vi "oa_Set Reset True If Parameters Change (N channels).vi"(6 "even angle position info":T1, 7 "reset? (T) in":bool=TRUE, 8 "FIR filter specifications in":T2={"alias rejection (dB)"=120.0, "normalized bandwidth"=0.4536} {"normalized bandwidth" format="%.4f"; "alias rejection (dB)" format="%.2f"}, 9 "interpolation mode in":u16(ring)=1 items=["coerce", "linear", "spline", "FIR filter"], 10 "dr in":dbl=1.0 format="%.2p", 11 "even angle signals":cluster{"r0":dbl, "dr":dbl, "Y":dbl[]}[](array[cluster]) {"r0" format="%.2p"; "dr" format="%.2p"; "Y" format="%.2f"}) -> (0 "FIR filter specifications out":T2={"alias rejection (dB)"=120.0, "normalized bandwidth"=0.4536} {"normalized bandwidth" format="%.4f"; "alias rejection (dB)" format="%.2f"}, 1 "interpolation mode out":u16(ring)=1 items=["coerce", "linear", "spline", "FIR filter"], 2 "dr out":dbl=1.0 format="%.2p", 3 "even angle signals out":cluster{"r0":dbl, "dr":dbl, "Y":dbl[]}[](array[cluster]) {"r0" format="%.2p"; "dr" format="%.2p"; "Y" format="%.2f"}, 4 "even angle position info out":T1, 5 "reset? (T) out":bool=TRUE)   [LabVIEW 2017, in "SoundVib_OAUtility.lvlib"]
uses:
  <vilib>/addons/Sound and Vibration/Order Analysis/Utility/SoundVib_OAUtility.lvlib
  <vilib>/addons/Sound and Vibration/Order Analysis/Misc/OAT Position Info.ctl
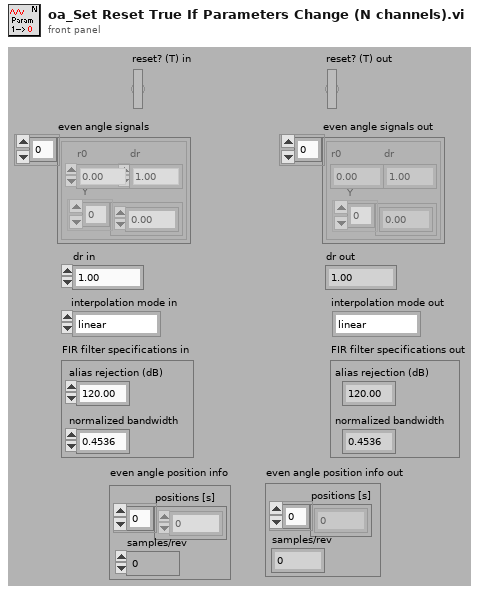
[diagram p1: front panel]
types:
  T1 = typedef "OAT Position Info.ctl" = cluster{"positions [s]":dbl[], "samples/rev":dbl}
  T2 = cluster{"alias rejection (dB)":dbl, "normalized bandwidth":dbl}
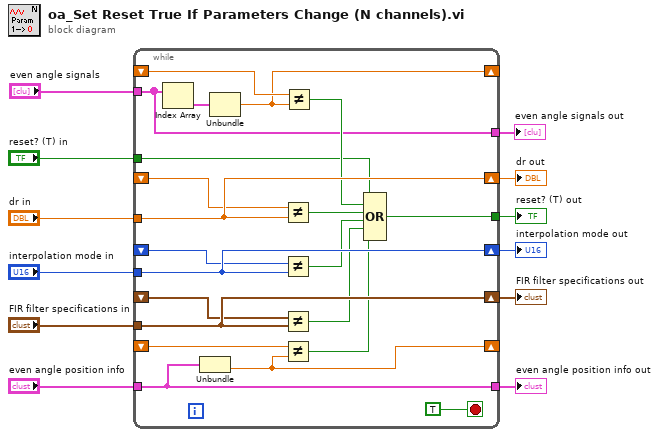
[diagram p0: block diagram]
diagram:
  n1 = while {
    tunnel: "dr in" -> [w32]
    shift-right: [w32] -> w7
    shift-left: _ -> [w31]
    tunnel: "interpolation mode in" -> [w30]
    shift-right: [w30] -> w6
    shift-left: _ -> [w29]
    tunnel: "FIR filter specifications in" -> [w28]
    shift-right: [w28] -> w5
    shift-left: _ -> [w27]
    tunnel: "even angle signals" -> [w17]
    shift-right: [w25] -> _
    shift-left: _ -> [w26]
    tunnel: "reset? (T) in" -> [w23]
    tunnel: [w19] -> w8
    tunnel: [w17] -> w3
    tunnel: "even angle position info" -> [w16]
    tunnel: [w16] -> w1
    shift-right: [w14] -> _
    shift-left: _ -> [w15]
    stop <- TRUE stop-if-true
    n2 = Index Array(array=w17) -> (element=w18:cluster{"r0":dbl, "dr":dbl, "Y":dbl[]})  [unwired: 1 in]
    n3 = Unbundle(w16) -> ("samples/rev"=w14:dbl)  [unwired: 1 out]
    n4 = Unbundle(w18) -> ("dr"=w25:dbl)  [unwired: 2 out]
    n5 = Not Equal?(x=w31, y=w32) -> (x != y?=w22:bool)
    n6 = Not Equal?(x=w29, y=w30) -> (x != y?=w21:bool)
    n7 = Not Equal?(x=w27, y=w28) -> (x != y?=w20:bool)
    n8 = Not Equal?(x=w15, y=w14) -> (x != y?=w13:bool)
    n9 = Not Equal?(x=w26, y=w25) -> (x != y?=w24:bool)
    n10 = Compound Arithmetic op=OR(w23, w24, w22, w21, w20, w13) -> (w19:bool)
  }
  "reset? (T) out" <- w8
  "dr out" <- w7
  "interpolation mode out" <- w6
  "FIR filter specifications out" <- w5
  "even angle signals out" <- w3
  "even angle position info out" <- w1
